vi "BinToDecimal.vi"(1 "Bin In":string) -> (0 "Decimal Out":u8)   [LabVIEW 2018]
panel:
  in  "cnt temp":u8
  out "length":i32
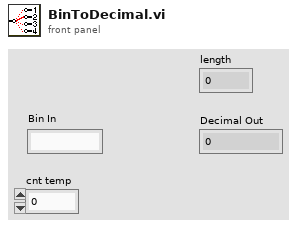
[diagram p1: front panel]
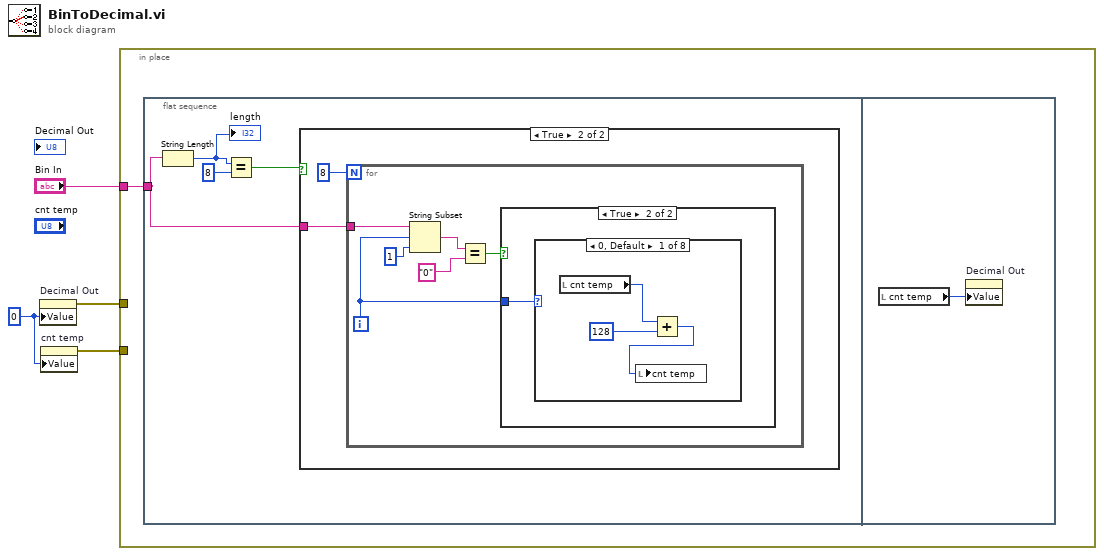
[diagram p0: block diagram]
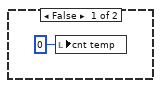
[diagram p2: hidden frame]
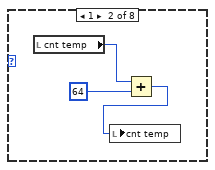
[diagram p4: hidden frame]
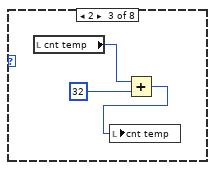
[diagram p5: hidden frame]
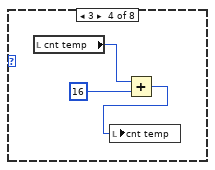
[diagram p6: hidden frame]
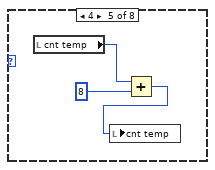
[diagram p7: hidden frame]
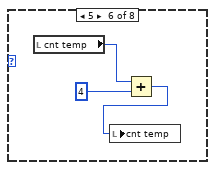
[diagram p8: hidden frame]
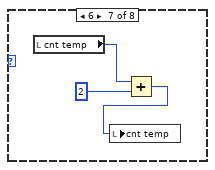
[diagram p9: hidden frame]
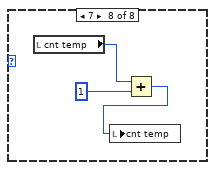
[diagram p10: hidden frame]
diagram:
  w2 = u8 0 ("Decimal Out")
  n1 = property on="Decimal Out" class="DigNum (strict)"("Value"=w2) -> (error out=w3:errorcluster)  [unwired: 2 in, 1 out]
  n2 = property on="cnt temp" class="DigNum (strict)"("Value"=w2) -> (error out=w1:errorcluster)  [unwired: 2 in, 1 out]
  n3 = in-place {
    in-place-border: "Bin In" -> [w5]
    in-place-border: w3 -> [_]
    in-place-border: w1 -> [_]
    n4 = flat-sequence {
      tunnel: w5 -> [w6]
      frame #0 {
        n5 = String Length(string=w6) -> (length=w9:i32)
        "length" <- w9
        n6 = Equal?(x=w9, y=8) -> (x = y?=w7:bool)
        n7 = case shown="True" w7 {
          tunnel: w6 -> [_ w11]
          frame False {
            n8 = local write "cnt temp"(u8 0 ("cnt temp")) -> ()
          }
          frame True {
            n9 = for {
              N: 8 -> [_]
              tunnel: w11 -> [w17]
              i -> [w13]
              n10 = String Subset(string=w17, offset (0)=w13, length (rest)=1 ("length (rest)")) -> (substring=w16:string)
              n11 = Equal?(x=w16, y="0") -> (x = y?=w14:bool)
              n12 = case shown="True" w14 {
                tunnel: w13 -> [_ w19]
                frame False {
                }
                frame True {
                  n13 = case shown="0, Default" w19 {
                    frame 0, Default {
                      n14 = local read "cnt temp"() -> (w22:u8)
                      n15 = Add(x=w22, y=u8 128) -> (x+y=w21:u8)
                      n16 = local write "cnt temp"(w21) -> ()
                    }
                    frame 1 {
                      n17 = local read "cnt temp"() -> (w25:u8)
                      n18 = Add(x=w25, y=u8 64) -> (x+y=w24:u8)
                      n19 = local write "cnt temp"(w24) -> ()
                    }
                    frame 2 {
                      n20 = local read "cnt temp"() -> (w28:u8)
                      n21 = Add(x=w28, y=u8 32) -> (x+y=w27:u8)
                      n22 = local write "cnt temp"(w27) -> ()
                    }
                    frame 3 {
                      n23 = local read "cnt temp"() -> (w31:u8)
                      n24 = Add(x=w31, y=u8 16) -> (x+y=w30:u8)
                      n25 = local write "cnt temp"(w30) -> ()
                    }
                    frame 4 {
                      n26 = local read "cnt temp"() -> (w34:u8)
                      n27 = Add(x=w34, y=u8 8) -> (x+y=w33:u8)
                      n28 = local write "cnt temp"(w33) -> ()
                    }
                    frame 5 {
                      n29 = local read "cnt temp"() -> (w37:u8)
                      n30 = Add(x=w37, y=u8 4) -> (x+y=w36:u8)
                      n31 = local write "cnt temp"(w36) -> ()
                    }
                    frame 6 {
                      n32 = local read "cnt temp"() -> (w40:u8)
                      n33 = Add(x=w40, y=u8 2) -> (x+y=w39:u8)
                      n34 = local write "cnt temp"(w39) -> ()
                    }
                    frame 7 {
                      n35 = local read "cnt temp"() -> (w43:u8)
                      n36 = Add(x=w43, y=u8 1) -> (x+y=w42:u8)
                      n37 = local write "cnt temp"(w42) -> ()
                    }
                  }
                }
              }
            }
          }
        }
      }
      frame #1 {
        n38 = local read "cnt temp"() -> (w44:u8)
        n39 = property on="Decimal Out" class="DigNum (strict)"("Value"=w44) -> ()  [unwired: 2 in, 2 out]
      }
    }
  }
